vi "Bardo's secret sauce for logarithmic drive.vi"(11 "Joystick Input":dbl) -> (3 "Scaled Output":dbl)   [LabVIEW 2017]
doc: "This subVI uses the logarithm base 2 of the input and gives the output."
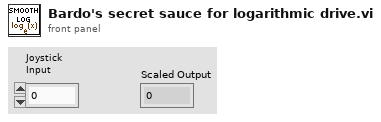
[diagram p1: front panel]
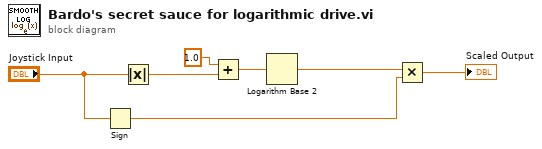
[diagram p0: block diagram]
diagram:
  n1 = Sign(1:"Joystick Input") -> (0:w4:dbl)
  n2 = Absolute Value(x="Joystick Input") -> (abs(x)=w1:dbl)
  n3 = Add(x=1.0, y=w1) -> (x+y=w7:dbl)
  n4 = Logarithm Base 2(1:w7) -> (0:w5:dbl)
  n5 = Multiply(x=w5, y=w4) -> (x*y=→"Scaled Output":dbl)
